vi "Configure Measurement.vi"(7 "Enable Auto Range (T:Enable)":bool=TRUE, 8 "error in (no error)":errorcluster, 9 "Manual Impedance Range (3: 100 Ohms)":i32(ring)=3 items=["100m", "1", "10", "100", "300", "1K", "3K", "10K", "30K", "100K"], 10 "Function (0: Cp-D)":u16(ring) items=["Cp-D", "Cp-Q", "Cp-G", "Cp-Rp", "Cs-D", "Cs-Q", "Cs-Rs", "Lp-D", "Lp-Q", "Lp-G", "Lp-Rp", "Lp-Rdc", "Ls-D", "Ls-Q", "Ls-Rs", "Ls-Rdc", "R-X", "Z-thd", "Z-thr", "G-B", "Y-thd", "Y-thr", "Vdc-Idc"], 11 "VISA resource name":refnum<visa-resource-name>) -> (0 "error out":errorcluster, 3 "VISA resource name out":refnum<visa-resource-name>)   [LabVIEW 2019, in "Agilent E4980.lvlib"]
doc: "Configures the measurement function and impedance range. The instrument simultaneously measures two components of the complex impedance (parameter) in a measurement cycle."
uses:
  Agilent E4980.lvlib
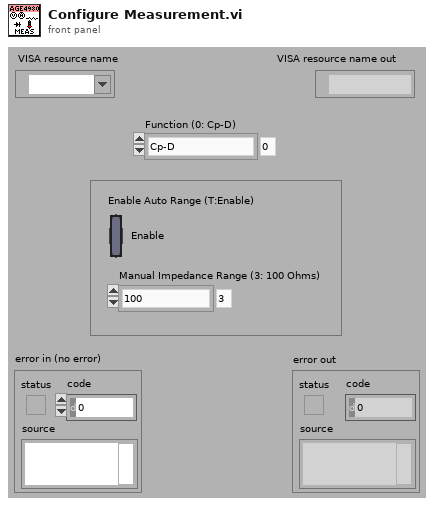
[diagram p1: front panel]
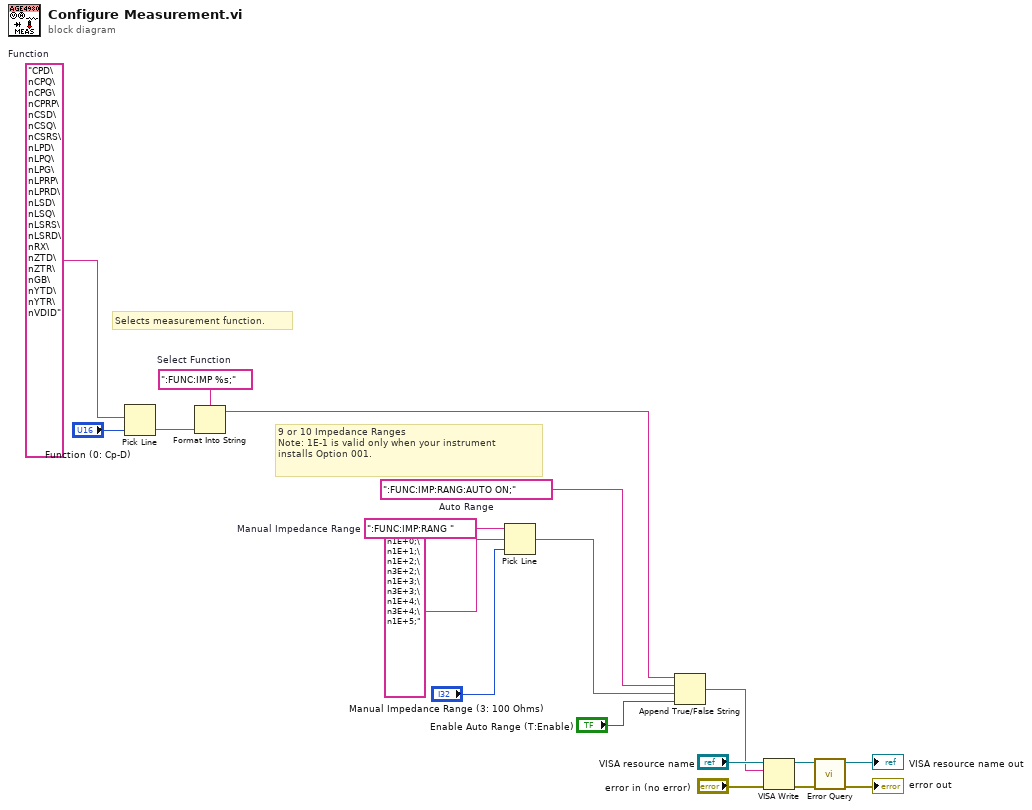
[diagram p0: block diagram]
diagram:
  w4 = ":FUNC:IMP:RANG "  # Manual Impedance Range
  w8 = ":FUNC:IMP:RANG:AUTO ON;"  # Auto Range
  w12 = ":FUNC:IMP %s;"  # Select Function
  w14 = "CPD\nCPQ\nCPG\nCPRP\nCSD\nCSQ\nCSRS\nLPD\nLPQ\nLPG\nLPRP\nLPRD\nLSD\nLSQ\nLSRS\nLSRD\nRX\nZTD\nZTR\nGB\nYTD\nYTR\nVDID"  # Function
  # "Selects measurement function."
  # "9 or 10 Impedance Ranges\nNote: 1E-1 is valid only when your instrument\ninstalls Option 001."
  n1 = Pick Line(multi-line string=w14, line index="Function (0: Cp-D)") -> (output string=w9:string)  [unwired: 1 in]
  n2 = Format Into String(format string=w12, w9) -> (resulting string=w6:string)  [unwired: 2 in, 1 out]
  n3 = Pick Line(string ("")=w4, multi-line string="1E-1;\n1E+0;\n1E+1;\n1E+2;\n3E+2;\n1E+3;\n3E+3;\n1E+4;\n3E+4;\n1E+5;", line index="Manual Impedance Range (3: 100 Ohms)") -> (output string=w1:string)
  n4 = Append True/False String(1:"Enable Auto Range (T:Enable)", 2:w1, 3:w8, 4:w6) -> (0:w5:string)
  n5 = VISA Write(VISA resource name="VISA resource name", write buffer=w5, error in (no error)="error in (no error)") -> (VISA resource name out=w11:refnum<visa-resource-name>, error out=w10:errorcluster)  [unwired: 1 out]
  n6 = call "Error Query.vi"("error in (no error)"=w10, "VISA resource name"=w11) -> ("error out"=→"error out":errorcluster, "VISA resource name out"=→"VISA resource name out":refnum<visa-resource-name>)  [unwired: 6 in, 2 out]
